vi "Test-DotNet-StatusMonitoring.vi"() -> ()   [LabVIEW 2013, in "EC1000-control.lvlib" / "SM1000-control.lvclass"]
uses:
  SM1000-control.lvclass
  DOTNET-settings.ctl
  Device-identification.ctl
  Status-information.ctl
  EC1000_DOTNET/getBroadcastData-status.vi
panel:
  out "Array":i16[][](array[numeric])
  in  "Period":u32
  out "EC1000 scan head commands":i16[][](graph)
  in  "Stop":bool
  out "serverList iterator":i32
  out "Status information":T1
  in  "Device index":i32
  out "piServerCount":i32
  out "Device identifiers":T2[](array[typedef])
  in  "DOTNET settings":T3={"Target IP"="128.178.146.163", "Target broadcast port"=11000, "Target communication port"=12200, "clientID"=-1, "Broadcast IP"="224.168.100.2", "Servercount"=-1, "Device IDs"=[]}
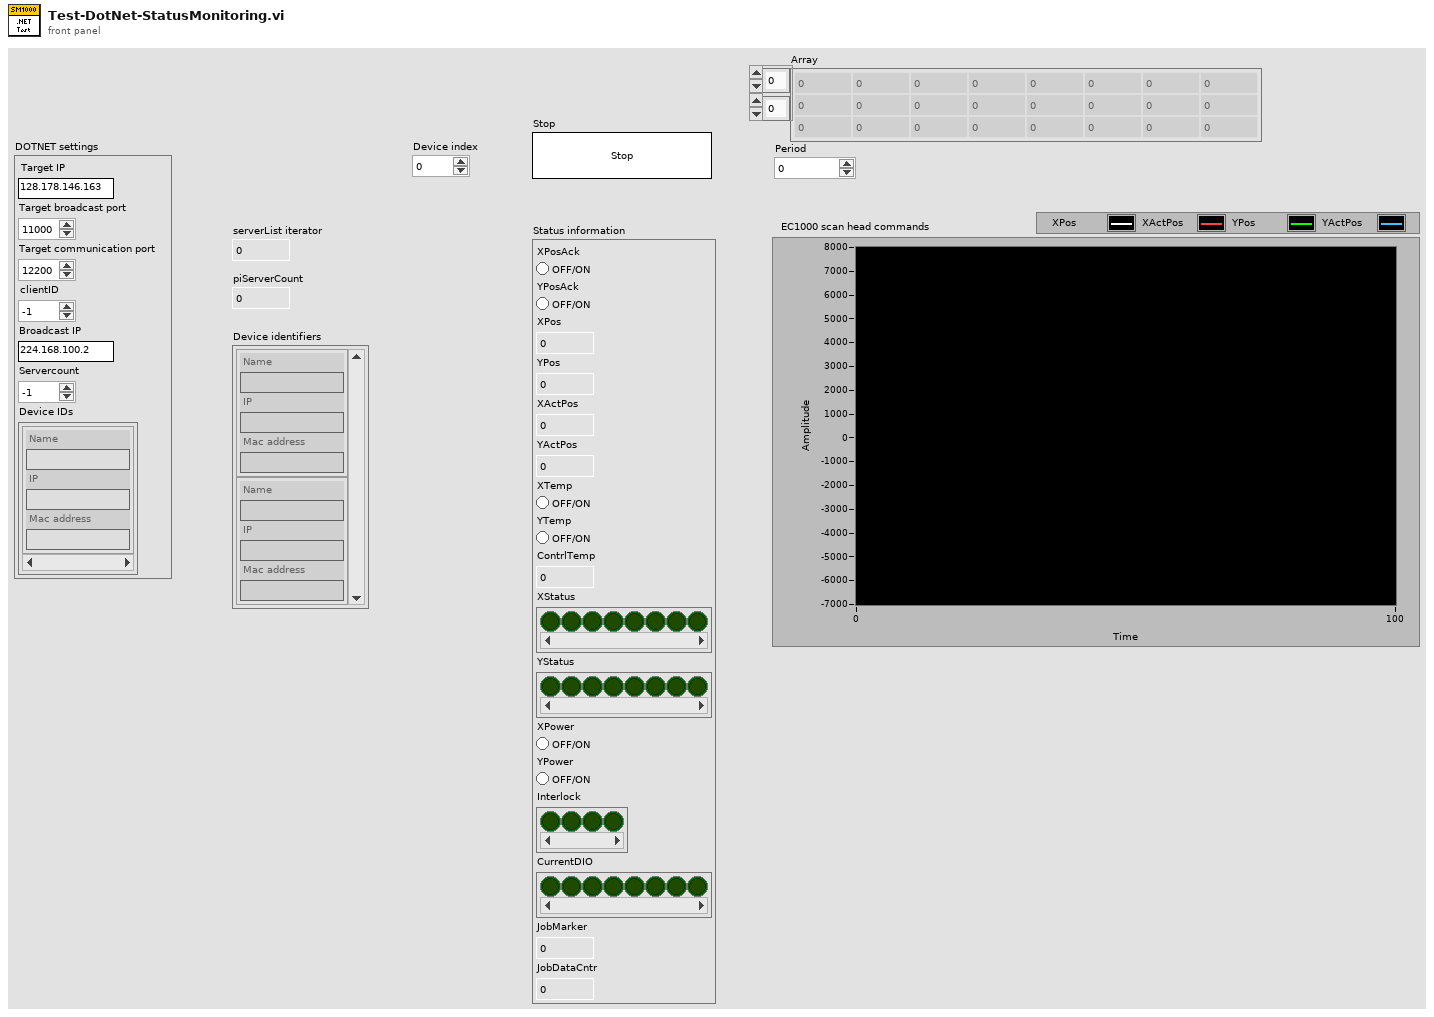
[diagram p1: front panel]
types:
  T1 = typedef "EC1000-control.lvlib/SM1000-control.lvclass/Status-information.ctl" = cluster{"XPosAck":bool, "YPosAck":bool, "XPos":i16, "YPos":i16, "XActPos":i16, "YActPos":i16, "XTemp":bool, "YTemp":bool, "ContrlTemp":i16, "XStatus":bool[], "YStatus":bool[], "XPower":bool, "YPower":bool, "Interlock":bool[], "CurrentDIO":bool[], "JobMarker":u16, "JobDataCntr":u32}
  T2 = typedef "EC1000-control.lvlib/SM1000-control.lvclass/Device-identification.ctl" = cluster{"Name":string, "IP":string, "Mac address":string}
  T3 = typedef "EC1000-control.lvlib/SM1000-control.lvclass/DOTNET-settings.ctl" = cluster{"Target IP":string, "Target broadcast port":i32, "Target communication port":i32, "clientID":i32, "Broadcast IP":string, "Servercount":i32, "Device IDs":T2[]}
  T4 = typedef "EC1000-control.lvlib/SM1000-control.lvclass/Object-reference.ctl" = refnum<data-value>
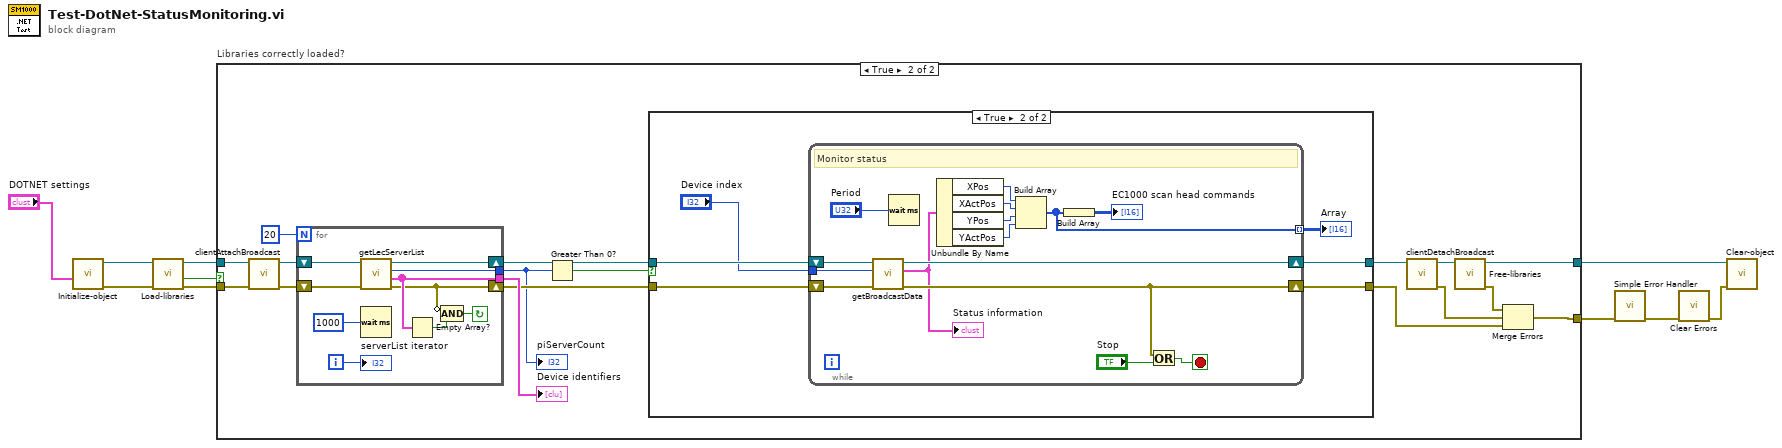
[diagram p0: block diagram]
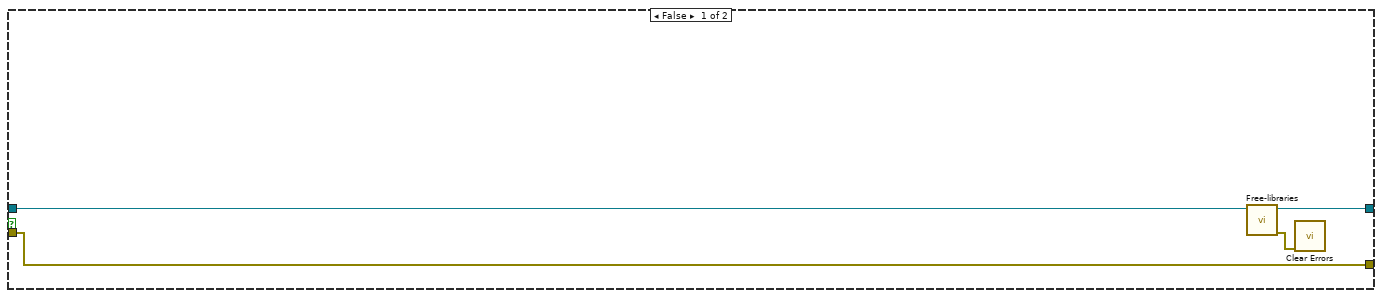
[diagram p2: hidden frame]
diagram:
  n1 = call "Initialize-object.vi"("DOTNET settings"="DOTNET settings") -> ("error out"=w8:errorcluster, "SM1000-control out"=w9:T4)  [unwired: 9 in]
  n2 = call "Load-libraries.vi"("error in (no error)"=w8, "SM1000-control in"=w9) -> ("error out"=w5:errorcluster, "Loaded?"=w7:bool, "SM1000-control out"=w6:T4)  [unwired: 7 in]
  n3 = case "Libraries correctly loaded?" shown="True" w7 {
    tunnel: w6 -> [w13 w28]
    tunnel: w5 -> [w14 w27]
    tunnel: [w14 w30] -> w3
    tunnel: [w12 w29] -> w1
    frame False {
      n4 = call "Free-libraries.vi"("SM1000-control in"=w13) -> ("error out"=w11:errorcluster, "SM1000-control out"=w12:T4)  [unwired: 8 in, 1 out]
      n5 = call <vilib>:"Clear Errors.vi"("error in (no error)"=w11) -> ()  [unwired: 6 in, 1 out]
    }
    frame True {
      n6 = call "clientAttachBroadcast.vi"("error in (no error)"=w27, "SM1000-control in"=w28) -> ("error out"=w23:errorcluster, "SM1000-control out"=w24:T4)  [unwired: 7 in, 1 out]
      n7 = for {
        N: 20 -> [_]
        tunnel: [w59] -> w22
        tunnel: [w62] -> w16
        shift-right: [w61] -> w18
        shift-left: w24 -> [w64]
        shift-right: [w56] -> w17
        shift-left: w23 -> [w63]
        i -> [w58]
        stop <- w55 continue-if-true
        n8 = call "getLecServerList.vi"("error in (no error)"=w63, "SM1000-control in"=w64) -> ("error out"=w56:errorcluster, "Device identifiers"=w59:T2[], "piServerCount"=w62:i32, "SM1000-control out"=w61:T4)  [unwired: 6 in]
        n9 = Wait (ms)(milliseconds to wait=u32 1000) -> ()  [unwired: 1 out]
        n10 = Empty Array?(array=w59) -> (empty?=w57:bool)
        n11 = Compound Arithmetic op=AND(invert w56, w57) -> (w55:bool)
        "serverList iterator" <- w58
      }
      "Device identifiers" <- w22
      "piServerCount" <- w16
      n12 = Greater Than 0?(x=w16) -> (x > 0?=w15:bool)
      n13 = case shown="True" w15 {
        tunnel: [w32 w35] -> w20
        tunnel: [w33 w36] -> w19
        tunnel: w18 -> [w33 w39]
        tunnel: w17 -> [w32 w38]
        frame False {
        }
        frame True {
          n14 = while {
            tunnel: "Device index" -> [w52]
            shift-right: [w51] -> w36
            shift-left: w39 -> [w54]
            shift-right: [w48] -> w35
            shift-left: w38 -> [w53]
            tunnel: [w40] -> w34 mode=indexing
            stop <- w50 stop-if-true
            # "Monitor status"
            n15 = call-poly "getBroadcastData.vi"("error in (no error)"=w53, "Device index"=w52, "SM1000-control in"=w54) -> ("error out"=w48:errorcluster, "Status information"=w47:T1, "SM1000-control out"=w51:T4)  [unwired: 6 in]
            "Status information" <- w47
            n16 = Wait (ms)(milliseconds to wait="Period") -> ()  [unwired: 1 out]
            n17 = Unbundle By Name(w47) -> ("XPos"=w44:i16, "XActPos"=w45:i16, "YPos"=w43:i16, "YActPos"=w42:i16)
            n18 = Build Array(w44, w45, w43, w42) -> (w40:i16[])
            n19 = Build Array(w40) -> (→"EC1000 scan head commands":i16[][])
            n20 = Or(x=w48, y="Stop") -> (x .or. y?=w50:bool)
          }
          "Array" <- w34
        }
      }
      n21 = call "clientDetachBroadcast.vi"("SM1000-control in"=w19) -> ("error out"=w25:errorcluster, "SM1000-control out"=w26:T4)  [unwired: 9 in]
      n22 = call "Free-libraries.vi"("SM1000-control in"=w26) -> ("error out"=w31:errorcluster, "SM1000-control out"=w29:T4)  [unwired: 8 in, 1 out]
      n23 = Merge Errors(w31, w25, w20) -> (w30:errorcluster)
    }
  }
  n24 = call <vilib>:"Simple Error Handler.vi"("error in (no error)"=w3) -> ("error out"=w4:errorcluster)  [unwired: 4 in, 4 out]
  n25 = call <vilib>:"Clear Errors.vi"("error in (no error)"=w4) -> ("error out"=w2:errorcluster)  [unwired: 6 in]
  n26 = call "Clear-object.vi"("error in (no error)"=w2, "SM1000-control"=w1) -> ()  [unwired: 8 in, 2 out]
